vi "Unreserve Sessions.vi"(8 "error in":errorcluster, 10 "sessions":T1[](array[typedef]), 11 "Measurement Context In":refnum<class "MeasurementContext.lvclass">) -> (0 "error out":errorcluster, 3 "Measurement Context Out":refnum<class "MeasurementContext.lvclass">)   [LabVIEW 2020, in "NIDCPowerSourceDCVoltage.lvlib"]
uses:
  <vilib>/MeasurementLink/MeasurementLink Session Management Client/RPC Messages/ni_measurementlink_sessionmanagement_v1_SessionInformation.ctl
  <vilib>/MeasurementLink/MeasurementLink Session Management Client/RPC Messages/nidevice_grpc_Session.ctl
  <vilib>/MeasurementLink/MeasurementLink Session Management Client/RPC Messages/ni_measurementlink_sessionmanagement_v1_ChannelMapping.ctl
  <vilib>/MeasurementLink/MeasurementLink Measurement Server/Classes/MeasurementContext/MeasurementContext.lvclass
  <vilib>/MeasurementLink/MeasurementLink Session Management Client/RPC Messages/ni_measurementlink_sessionmanagement_v1_UnreserveSessionsRequest.ctl
  <vilib>/MeasurementLink/MeasurementLink Measurement Server/Classes/MeasurementContext/MeasurementContext.lvclass/MeasurementContext.ctl
  <vilib>/MeasurementLink/MeasurementLink Measurement Server/Classes/MeasurementContext/Accessor/Read Session manager service gRPC ID.vi
  <vilib>/MeasurementLink/MeasurementLink Measurement Server/Classes/MeasurementContext/Accessor/Read Discovery service gRPC ID.vi
  NIDCPowerSourceDCVoltage.lvlib
  <vilib>/MeasurementLink/MeasurementLink Discovery Client/MeasurementLink Discovery Client.lvlib
  <vilib>/MeasurementLink/MeasurementLink Session Management Client/MeasurementLink Session Management Client.lvlib
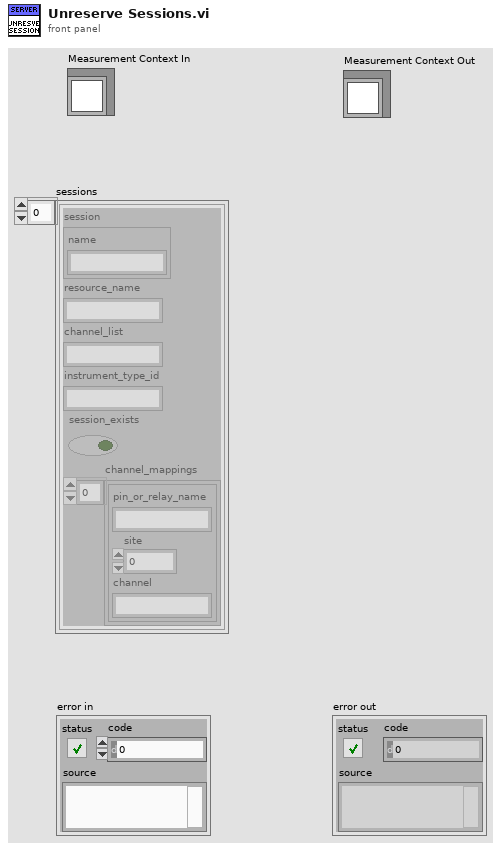
[diagram p1: front panel]
types:
  T1 = typedef "MeasurementLink Session Management Client.lvlib/ni_measurementlink_sessionmanagement_v1_SessionInformation.ctl" = cluster{"session":T2, "resource_name":string, "channel_list":string, "instrument_type_id":string, "session_exists":bool, "channel_mappings":T3[]}
  T2 = typedef "MeasurementLink Session Management Client.lvlib/nidevice_grpc_Session.ctl" = cluster{"name":string}
  T3 = typedef "MeasurementLink Session Management Client.lvlib/ni_measurementlink_sessionmanagement_v1_ChannelMapping.ctl" = cluster{"pin_or_relay_name":string, "site":i32, "channel":string}
  T4 = typedef "MeasurementLink Session Management Client.lvlib/ni_measurementlink_sessionmanagement_v1_UnreserveSessionsRequest.ctl" = cluster{"sessions":T1[]}
  T5 = typedef "grpc-lvsupport-release.lvlib/grpcId.ctl" = u64
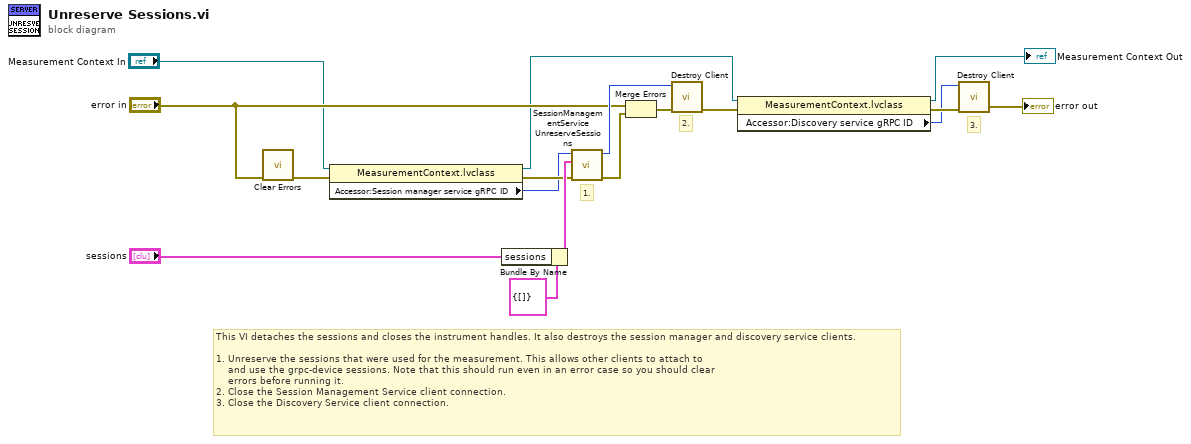
[diagram p0: block diagram]
diagram:
  # "This VI detaches the sessions and closes the instrument handles. It also destroys the session manager and discovery service clients.\n\n1. Unreserve the sessions that were used for the measurement. This allows other clients to attach to\n    and use the grpc-device sessions. Note that this should run even in an error case so you should clear \n    errors before running it.\n2. Close the Session Management Service client connection.\n3. Close the Discovery Service client connection."
  # "1."
  # "3."
  # "2."
  n1 = call <vilib>:"Clear Errors.vi"("error in (no error)"="error in") -> ("error out"=w15:errorcluster)  [unwired: 5 in, 1 out]
  n2 = property class="MeasurementContext.lvclass"(reference="Measurement Context In", error in=w15) -> (reference out=w3:refnum<class "MeasurementContext.lvclass">, error out=w7:errorcluster, "Accessor:Session manager service gRPC ID"=w5:T5)
  n3 = Bundle By Name(cluster=T4 {"sessions"=[]} ("Request Data"), "sessions"="sessions") -> (w13:T4)
  n4 = call <vilib>:"SessionManagementService UnreserveSessions.vi"("error in"=w7, "Request Data"=w13, "gRPC ID"=w5) -> ("error out"=w11:errorcluster, "gRPC ID out"=w17:T5)  [unwired: 6 in, 1 out]
  n5 = Merge Errors("error in", w11) -> (w12:errorcluster)
  n6 = call <vilib>:"Destroy Client.vi"("error in"=w12, "gRPC ID"=w17) -> ("error out"=w16:errorcluster)  [unwired: 9 in]
  n7 = property class="MeasurementContext.lvclass"(reference=w3, error in=w16) -> (reference out=→"Measurement Context Out":refnum<class "MeasurementContext.lvclass">, error out=w4:errorcluster, "Accessor:Discovery service gRPC ID"=w2:T5)
  n8 = call <vilib>:"Destroy Client.vi"("error in"=w4, "gRPC ID"=w2) -> ("error out"=→"error out":errorcluster)  [unwired: 9 in]
